vi "PointToSetting_um.vi"(10 "Clicked":dbl[](array[numeric]), 11 "Scan Settings":T1) -> (3 "Setting":dbl[](array[numeric]))   [LabVIEW 2014]
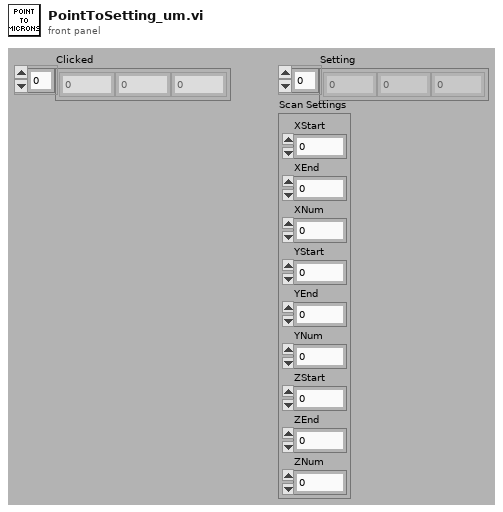
[diagram p1: front panel]
types:
  T1 = cluster{"XStart":dbl, "XEnd":dbl, "XNum":dbl, "YStart":dbl, "YEnd":dbl, "YNum":dbl, "ZStart":dbl, "ZEnd":dbl, "ZNum":dbl}
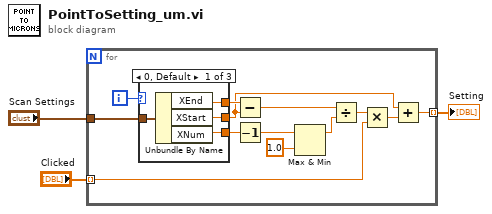
[diagram p0: block diagram]
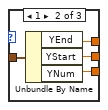
[diagram p2: hidden frame]
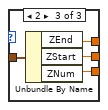
[diagram p3: hidden frame]
diagram:
  n1 = for {
    tunnel: "Clicked" -> [w12] mode=indexing
    tunnel: "Scan Settings" -> [w16]
    tunnel: [w9] -> w2 mode=indexing
    i -> [w15]
    n2 = case shown="0, Default" w15 {
      tunnel: w16 -> [w20 w24 w28]
      tunnel: [w19 w23 w27] -> w13
      tunnel: [w18 w22 w26] -> w10
      tunnel: [w17 w21 w25] -> w8
      frame 0, Default {
        n3 = Unbundle By Name(w20) -> ("XEnd"=w19:dbl, "XStart"=w18:dbl, "XNum"=w17:dbl)
      }
      frame 1 {
        n4 = Unbundle By Name(w24) -> ("YEnd"=w23:dbl, "YStart"=w22:dbl, "YNum"=w21:dbl)
      }
      frame 2 {
        n5 = Unbundle By Name(w28) -> ("ZEnd"=w27:dbl, "ZStart"=w26:dbl, "ZNum"=w25:dbl)
      }
    }
    n6 = Subtract(x=w13, y=w10) -> (x-y=w14:dbl)
    n7 = Decrement(x=w8) -> (x-1=w5:dbl)
    n8 = Max & Min(x=w5, y=1.0) -> (max(x,y)=w4:dbl)  [unwired: 1 out]
    n9 = Divide(x=w14, y=w4) -> (x/y=w7:dbl)
    n10 = Multiply(x=w7, y=w12) -> (x*y=w11:dbl)
    n11 = Add(x=w10, y=w11) -> (x+y=w9:dbl)
  }
  "Setting" <- w2
